vi "FTP (SubVI).vi"(8 "error in":errorcluster, 11 "semaphore":T1) -> (0 "error IO":errorcluster, 3 "semaphore out":T1)   [LabVIEW 2015]
uses:
  <vilib>/FTP/NI_FTP.lvlib
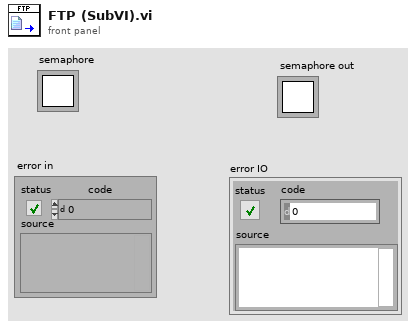
[diagram p1: front panel]
types:
  T1 = typedef "Semaphore RefNum" = refnum<k1>
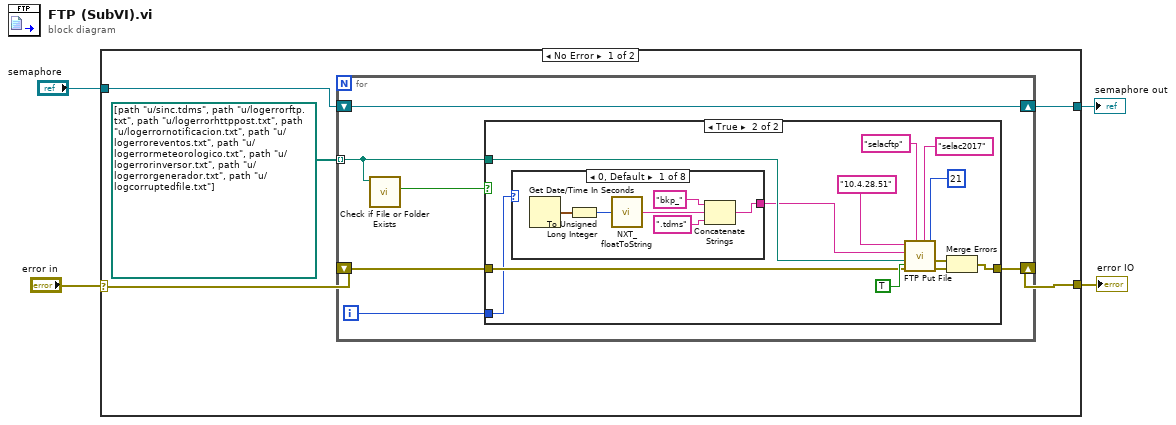
[diagram p0: block diagram]
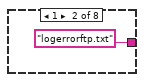
[diagram p3: hidden frame]
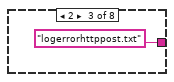
[diagram p4: hidden frame]
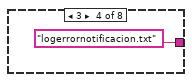
[diagram p5: hidden frame]
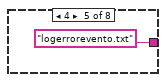
[diagram p6: hidden frame]
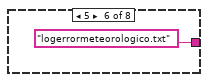
[diagram p7: hidden frame]
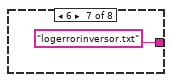
[diagram p8: hidden frame]
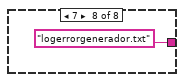
[diagram p9: hidden frame]
diagram:
  n1 = case shown="No Error" "error in" {
    selector: "error in" -> [w9 w43]
    tunnel: [w8 w43] -> w3
    tunnel: [w7 w42] -> w2
    tunnel: "semaphore" -> [w6 w42]
    frame No Error {
      n2 = for {
        shift-right: [w15] -> w8
        shift-left: w9 -> [w13]
        tunnel: path[] [path "u:/sinc.tdms", path "u:/logerrorftp.txt", path "u:/logerrorhttppost.txt", path "u:/logerrornotificacion.txt", path "u:/logerroreventos.txt", path "u:/logerrormeteorologico.txt", path "u:/logerrorinversor.txt", path "u:/logerrorgenerador.txt", path "u:/logcorruptedfile.txt"] -> [w10] mode=indexing
        shift-right: [w14] -> w7
        shift-left: w6 -> [w14]
        i -> [w12]
        n3 = call <vilib>:"Check if File or Folder Exists.vi"("path"=w10) -> ("file or folder exists?"=w11:bool)  [unwired: 8 in, 2 out]
        n4 = case shown="True" w11 {
          tunnel: [w16 w21] -> w15
          tunnel: w10 -> [_ w20]
          tunnel: w13 -> [w16 w18]
          tunnel: w12 -> [_ w17]
          frame False {
          }
          frame True {
            n5 = case shown="0, Default" w17 {
              tunnel: [w29 "logerrorftp.txt" "logerrorhttppost.txt" "logerrornotificacion.txt" "logerrorevento.txt" "logerrormeteorologico.txt" "logerrorinversor.txt" "logerrorgenerador.txt"] -> w19
              frame 0, Default {
                n6 = Get Date/Time In Seconds() -> (seconds since 1Jan1904=w31:timestamp)
                n7 = To Unsigned Long Integer(number=w31) -> (unsigned 32bit integer=w32:u32)
                n8 = call <vilib>:"NXT_floatToString.vi"("number"=w32) -> ("string"=w33:string)
                n9 = Concatenate Strings("bkp_" ("remote path"), w33, ".tdms" ("string")) -> (w29:string)
              }
              frame 1 {
              }
              frame 2 {
              }
              frame 3 {
              }
              frame 4 {
              }
              frame 5 {
              }
              frame 6 {
              }
              frame 7 {
              }
            }
            n10 = call <vilib>:"FTP Put File.vi"("remote port (21)"=u16 21, "password"="selac2017", "binary (F)"=TRUE, "user"="selacftp", "error in (no error)"=w18, "local path"=w20, "remote path"=w19, "host"="10.4.28.51") -> ("error out"=w22:errorcluster, "file error"=w23:errorcluster)  [unwired: 2 in]
            n11 = Merge Errors(w23, w22) -> (w21:errorcluster)
          }
        }
      }
    }
    frame Error {
    }
  }
  "error IO" <- w3
  "semaphore out" <- w2
